vi "saveFile.vi"(11 "path":path) -> ()   [LabVIEW 2016]
uses:
  variables/imageSettings.vi
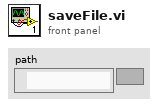
[diagram p1: front panel]
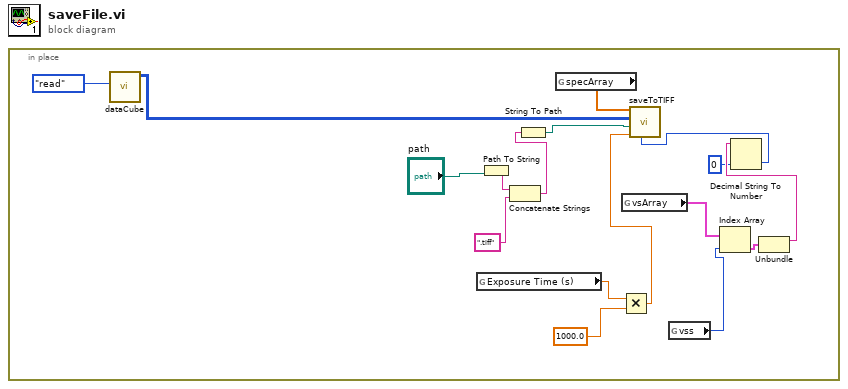
[diagram p0: block diagram]
diagram:
  n1 = in-place {
    n2 = call "dataCube.vi"("Enum"=enum16{"clear", "read", "write"}."read") -> ("imageCubeOut"=w1:i32[][][])  [unwired: 8 in, 2 out]
    n3 = global read "imageSettings.vi" "Exposure Time (s)"() -> (w6:sgl)
    n4 = Path To String(path="path") -> (string=w16:string)
    n5 = Concatenate Strings(w16, ".tiff" ("string")) -> (w15:string)
    n6 = String To Path(string=w15) -> (path=w12:path)
    n7 = global read "imageSettings.vi" "specArray"() -> (w5:sgl[])
    n8 = Multiply(x=w6, y=sgl 1000.0) -> (x*y=w11:sgl)
    n9 = global read "imageSettings.vi" "vsArray"() -> (w2:cluster{"String":string, "Value":u16}[])
    n10 = global read "imageSettings.vi" "vss"() -> (w3:i32)
    n11 = Index Array(array=w2, index=w3) -> (element=w10:cluster{"String":string, "Value":u16})
    n12 = Unbundle(w10) -> ("String"=w9:string)  [unwired: 1 out]
    n13 = Decimal String To Number(string=w9, default (0L)=u16 0 ("default (0 I32)")) -> (number=w8:u16)  [unwired: 1 in, 1 out]
    n14 = call "saveToTIFF.vi"("SPEC.CCD.Andor.VSS"=w8, "SPEC.CCD.Exposure(ms )"=w11, "selected path"=w12, "Array"=w1, "x array"=w5) -> ()  [unwired: 7 in]
  }
